vi "抓邊_線.vi"(0 "Image In":T4, 1 "Process":T8(ring), 2 "Optimized Mode":bool, 5 "ROI":T6, 7 "Options":T3={"Search Direction"=0, "Edge Options"={"Edge Polarity"=0, "Kernel Size"=3, "Width"=3, "Minimum Edge Strength"=10.0, "Interpolation Type"=enum."Bilinear Fixed", "Data Processing Method"=enum."Average"}, "Show Search Area"=FALSE, "Show Search Lines"=FALSE, "Show Edges Found"=FALSE, "Show Result"=TRUE, "Search Area Color"=65280, "Search Lines Color"=255, "Edge Locations Color"=16776960, "Result Color"=16711680, "Overlay Group Name"=""} {"Edge Options"."Edge Polarity" items=["All Edges", "Rising Edges", "Falling Edges"]; "Edge Options"."Minimum Edge Strength" format="%.2f"; "Edge Options"."Width" step=2; "Edge Options"."Kernel Size" step=2; "Search Direction" items=["Start to End", "End to Start"]}, 11 "error In":errorcluster, 13 "Point Diameter (5)":u32=5 min=3 max=1000) -> (4 "Image Out":T4, 6 "Line Profile":T7(graph), 10 "Gradient Information":dbl[][](graph), 14 "Location (Pixel)":cluster{"X":sgl, "Y":sgl}, 15 "error out":errorcluster)   [LabVIEW 2015]
uses:
  <vilib>/vision/Image Controls.llb/IMAQ Image.ctl
  <vilib>/vision/Measure.llb/Edge Options.ctl
  <vilib>/vision/Measure.llb/Edge Polarity.ctl
  <vilib>/vision/NI_Vision_Development_Module.lvlib
panel:
  out "Line":T5 {"Start X" scale=0.0..1024.0; "End X" scale=0.0..1024.0}
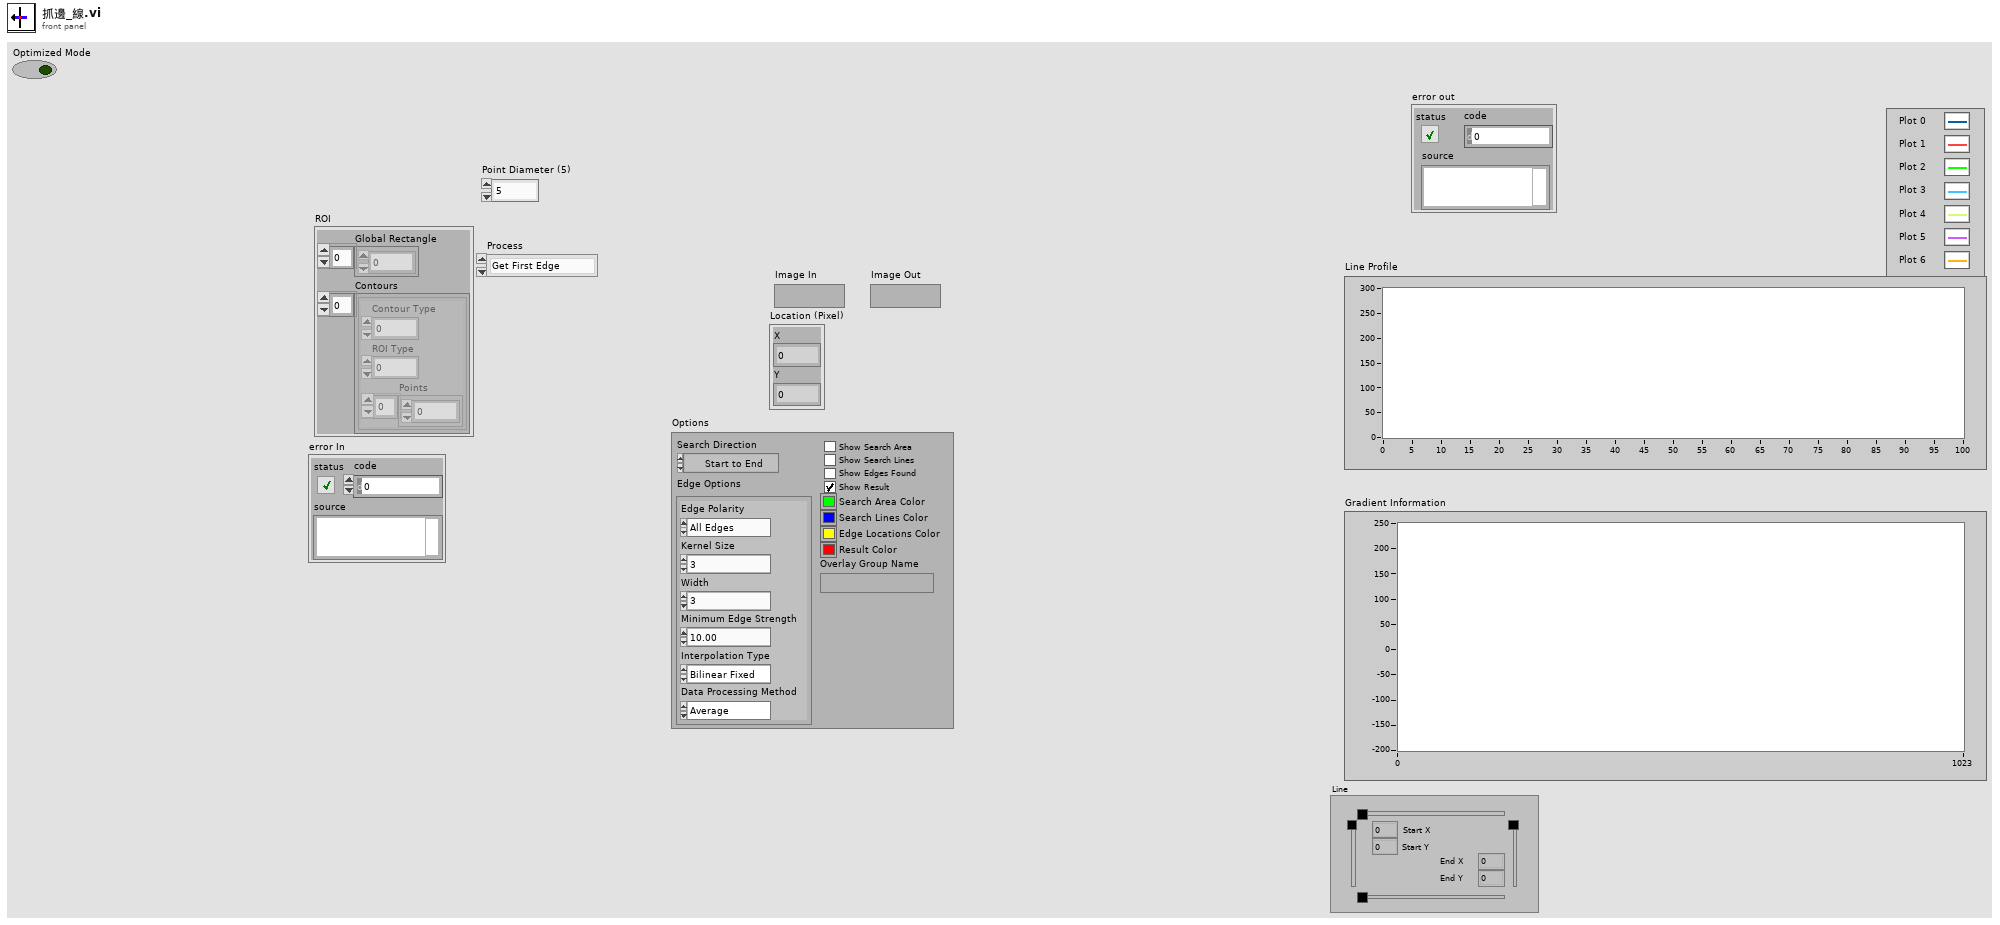
[diagram p1: front panel]
types:
  T1 = typedef "Edge Options.ctl" = cluster{"Edge Polarity":T2, "Kernel Size":u32, "Width":u32, "Minimum Edge Strength":sgl, "Interpolation Type":enum32{"Zero Order", "Bilinear", "Quadratic", "Cubic", "Bilinear Fixed"}, "Data Processing Method":enum32{"Average", "Median"}}
  T2 = typedef "Edge Polarity.ctl" = u32
  T3 = cluster{"Search Direction":u32, "Edge Options":T1, "Show Search Area":bool, "Show Search Lines":bool, "Show Edges Found":bool, "Show Result":bool, "Search Area Color":u32, "Search Lines Color":u32, "Edge Locations Color":u32, "Result Color":u32, "Overlay Group Name":string}
  T4 = typedef "IMAQ Image.ctl" = refnum<image>
  T5 = typedef "IMAQ Line" = cluster{"Start X":i32, "Start Y":i32, "End X":i32, "End Y":i32}
  T6 = cluster{"Global Rectangle":i32[], "Contours":cluster{"Contour Type":u32, "ROI Type":u32, "Points":i32[]}[]}
  T7 = cluster{"x0":sgl, "dx":sgl, "Pixels Line":sgl[]}[]
  T8 = enum16{"Get First Edge", "Get First + Last Edge", "Get All Edges", "Get Best Edge"}
  T9 = cluster{"Point 1":cluster{"x":dbl, "y":dbl}, "Point 2":cluster{"x":dbl, "y":dbl}}
  T10 = typedef "ROI Descriptor" = cluster{"Global Rectangle":i32[], "Contours":cluster{"ID":enum32{"External", "Internal"}, "Type":u32, "Coordinates":i32[]}[]}
  T11 = typedef "Edge New.ctl" = cluster{"Location (Pixel)":cluster{"X":sgl, "Y":sgl}, "Location (Real-World)":cluster{"X":sgl, "Y":sgl}, "Distance (Pixel)":dbl, "Distance (Real-World)":dbl, "Strength":dbl, "Noise":dbl, "Rising?":bool}
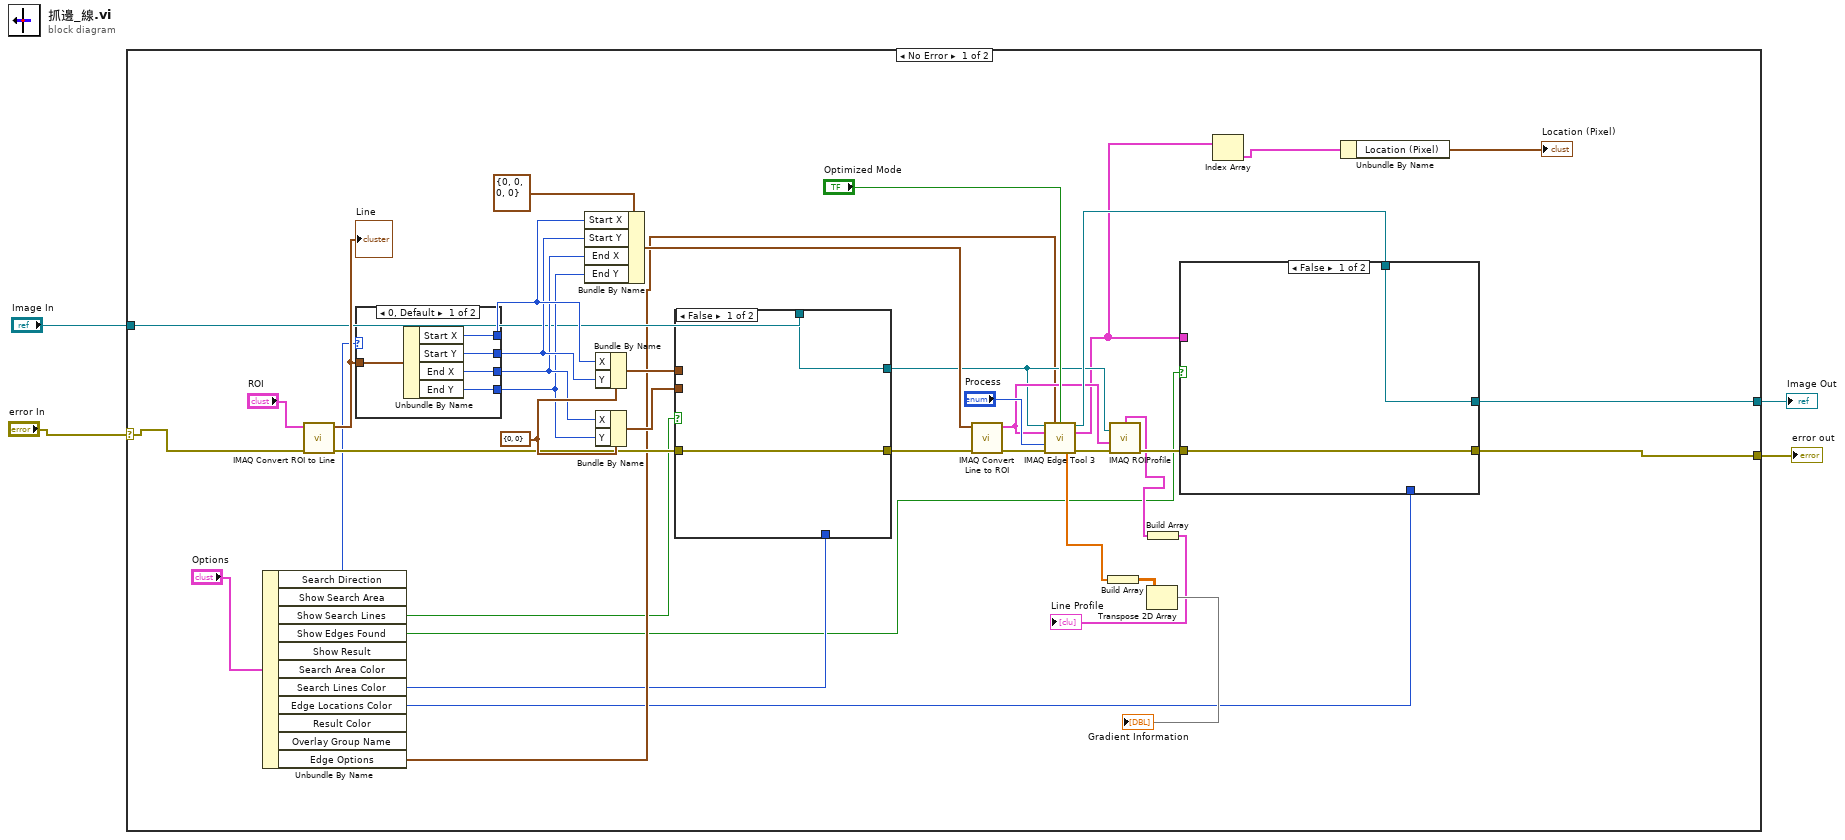
[diagram p0: block diagram]
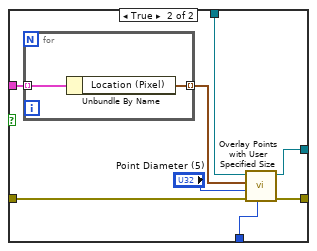
[diagram p2: hidden frame]
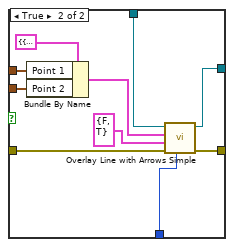
[diagram p3: hidden frame]
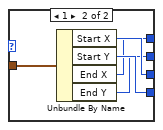
[diagram p4: hidden frame]
diagram:
  n1 = case shown="No Error" "error In" {
    selector: "error In" -> [w6 w79]
    tunnel: [w42 w79] -> w4
    tunnel: "Image In" -> [w23 w80]
    tunnel: [w22 w80] -> w2
    frame No Error {
      w30 = cluster{"X":i32, "Y":i32} {"X"=0, "Y"=0} ("Start Point")
      n2 = Unbundle By Name("Options") -> ("Search Direction"=w5:u32, "Show Search Lines"=w10:bool, "Show Edges Found"=w8:bool, "Search Lines Color"=w9:u32, "Edge Locations Color"=w7:u32, "Edge Options"=w11:T1)  [unwired: 5 out]
      n3 = call "IMAQ Convert ROI to Line"("error in (no error)"=w6, "ROI Descriptor"="ROI") -> ("error out"=w21:errorcluster, "Line"=w43:T5)  [unwired: 7 in]
      "Line" <- w43
      n4 = case shown="0, Default" w5 {
        tunnel: w43 -> [w73 w74]
        tunnel: [w72 w76] -> w28
        tunnel: [w71 w75] -> w27
        tunnel: [w70 w78] -> w26
        tunnel: [w69 w77] -> w25
        frame 0, Default {
          n5 = Unbundle By Name(w73) -> ("Start X"=w72:i32, "Start Y"=w71:i32, "End X"=w70:i32, "End Y"=w69:i32)
        }
        frame 1 {
          n6 = Unbundle By Name(w74) -> ("Start X"=w78:i32, "Start Y"=w77:i32, "End X"=w76:i32, "End Y"=w75:i32)
        }
      }
      n7 = Bundle By Name(cluster=T5 {"Start X"=0, "Start Y"=0, "End X"=0, "End Y"=0} ("Line"), "Start X"=w28, "Start Y"=w27, "End X"=w26, "End Y"=w25) -> (w34:T5)
      n8 = Bundle By Name(cluster=w30, "X"=w28, "Y"=w27) -> (w31:cluster{"X":i32, "Y":i32})
      n9 = Bundle By Name(cluster=w30, "X"=w26, "Y"=w25) -> (w29:cluster{"X":i32, "Y":i32})
      n10 = case shown="False" w10 {
        tunnel: [w58 w65] -> w33
        tunnel: [w57 w64] -> w32
        tunnel: w31 -> [_ w63]
        tunnel: w29 -> [_ w62]
        tunnel: w23 -> [w58 w61]
        tunnel: w21 -> [w57 w60]
        tunnel: w9 -> [_ w59]
        frame False {
        }
        frame True {
          n11 = Bundle By Name(cluster=T9 {"Point 1"={"x"=50.0, "y"=50.0}, "Point 2"={"x"=70.0, "y"=70.0}} ("Line Coordinates"), "Point 1"=w63, "Point 2"=w62) -> (w66:T9)
          n12 = call "Overlay Line with Arrows Simple.vi"("Color"=w59, "error in"=w60, "Arrows"=cluster{"Start point":bool, "End point":bool} {"Start point"=FALSE, "End point"=TRUE}, "Line Coordinates"=w66, "Image In"=w61) -> ("error out"=w64:errorcluster, "Image Out"=w65:T4)  [unwired: 5 in]
        }
      }
      n13 = call "IMAQ Convert Line to ROI"("error in (no error)"=w32, "Line"=w34) -> ("error out"=w37:errorcluster, "ROI Descriptor"=w36:T10)  [unwired: 7 in]
      n14 = call "IMAQ Edge Tool 3"("Image"=w33, "Edge Options"=w11, "Optimized Mode"="Optimized Mode", "ROI Descriptor"=w36, "Process"="Process", "error in (no error)"=w37) -> ("Image (duplicate)"=w39:T4, "Edge Information"=w17:T11[], "Gradient Values"=w20:dbl[], "error out"=w38:errorcluster)  [unwired: 5 in, 1 out]
      n15 = Build Array(w20) -> (w19:dbl[][])
      n16 = call "IMAQ ROIProfile"("error in (no error)"=w38, "ROI Descriptor"=w36, "Image"=w33) -> ("error out"=w41:errorcluster, "ROI Graph"=w14:cluster{"x0":sgl, "dx":sgl, "Pixels Line":sgl[]})  [unwired: 1 in, 3 out]
      n17 = Transpose 2D Array(2D array=w19) -> (transposed array=→"Gradient Information":dbl[][])
      n18 = Build Array(w14) -> (→"Line Profile":T7)
      n19 = case shown="False" w8 {
        tunnel: [w45 w54] -> w42
        tunnel: w41 -> [w45 w53]
        tunnel: w39 -> [w46 w52]
        tunnel: [w46 w49] -> w22
        tunnel: w17 -> [_ w48]
        tunnel: w7 -> [_ w47]
        frame False {
        }
        frame True {
          n20 = for {
            tunnel: w48 -> [w56] mode=indexing
            tunnel: [w55] -> w51 mode=indexing
            n21 = Unbundle By Name(w56) -> ("Location (Pixel)"=w55:cluster{"X":sgl, "Y":sgl})
          }
          n22 = call "Overlay Points with User Specified Size.vi"("Color"=w47, "error in"=w53, "Point Diameter (5)"="Point Diameter (5)", "Points"=w51, "Image In"=w52) -> ("error out"=w54:errorcluster, "Image Out"=w49:T4)  [unwired: 5 in]
        }
      }
      n23 = Index Array(array=w17) -> (element=w16:T11)  [unwired: 1 in]
      n24 = Unbundle By Name(w16) -> ("Location (Pixel)"=→"Location (Pixel)":cluster{"X":sgl, "Y":sgl})
    }
    frame Error {
    }
  }
  "Image Out" <- w2
  "error out" <- w4
